vi "VIServer_StopAllVIs.vi"() -> ()   [LabVIEW 2016]
panel:
  out "数组":string[](array[string])
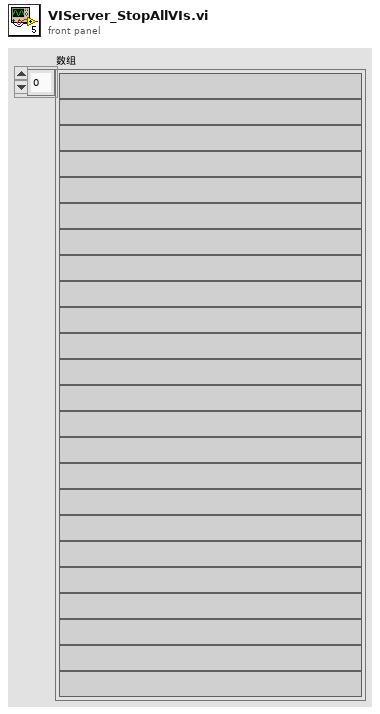
[diagram p1: front panel]
types:
  T1 = enum32{"Bad", "Idle", "Run top level", "Running"}
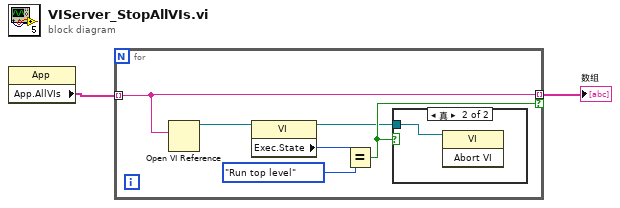
[diagram p0: block diagram]
diagram:
  n1 = property class="App"() -> ("App.AllVIs"=w2:string[])  [unwired: 2 in, 2 out]
  n2 = for {
    tunnel: w2 -> [w5] mode=indexing
    tunnel: [w5] -> w1 mode=indexing if=w4
    n3 = Open VI Reference(vi path=w5) -> (vi reference=w8:refnum<vi>)  [unwired: 5 in, 1 out]
    n4 = property class="VI"(reference=w8) -> (reference out=w3:refnum<vi>, "Exec.State"=w7:T1)  [unwired: 1 in, 1 out]
    n5 = Equal?(x=w7, y=T1."Run top level") -> (x = y?=w4:bool)
    n6 = case shown="真" w4 {
      tunnel: w3 -> [_ w9]
      frame False {
      }
      frame True {
        n7 = invoke class="VI" method="Abort VI"(reference=w9) -> ()  [unwired: 2 in, 3 out]
      }
    }
  }
  "数组" <- w1
